vi "BTS_PWMTest_GDCB-7_v1.vi"(8 "error in (no error)":errorcluster, 10 "HMP VISA":refnum<visa-resource-name>, 11 "ControlBoard VISA":refnum<visa-resource-name>) -> (0 "error out":errorcluster, 2 "Message OUT":string, 3 "Result (bool)":bool)   [LabVIEW 2022 SP3]
uses:
  HMP4000 Communication/HMP4040_ChannelControlAutomatic.ctl
  <vilib>/DAQmx/read.llb/DAQmx Read (Analog 1D Wfm NChan NSamp).vi
  <vilib>/DAQmx/miscellaneous.llb/DAQmx Fill In Error Info.vi
panel:
  in  "Message IN":string=" "
  out "Analysis Leg":i32
  out "Waveforms":T1
  out "Active Leg":i32
  out "Result (color)":u32(colorbox)
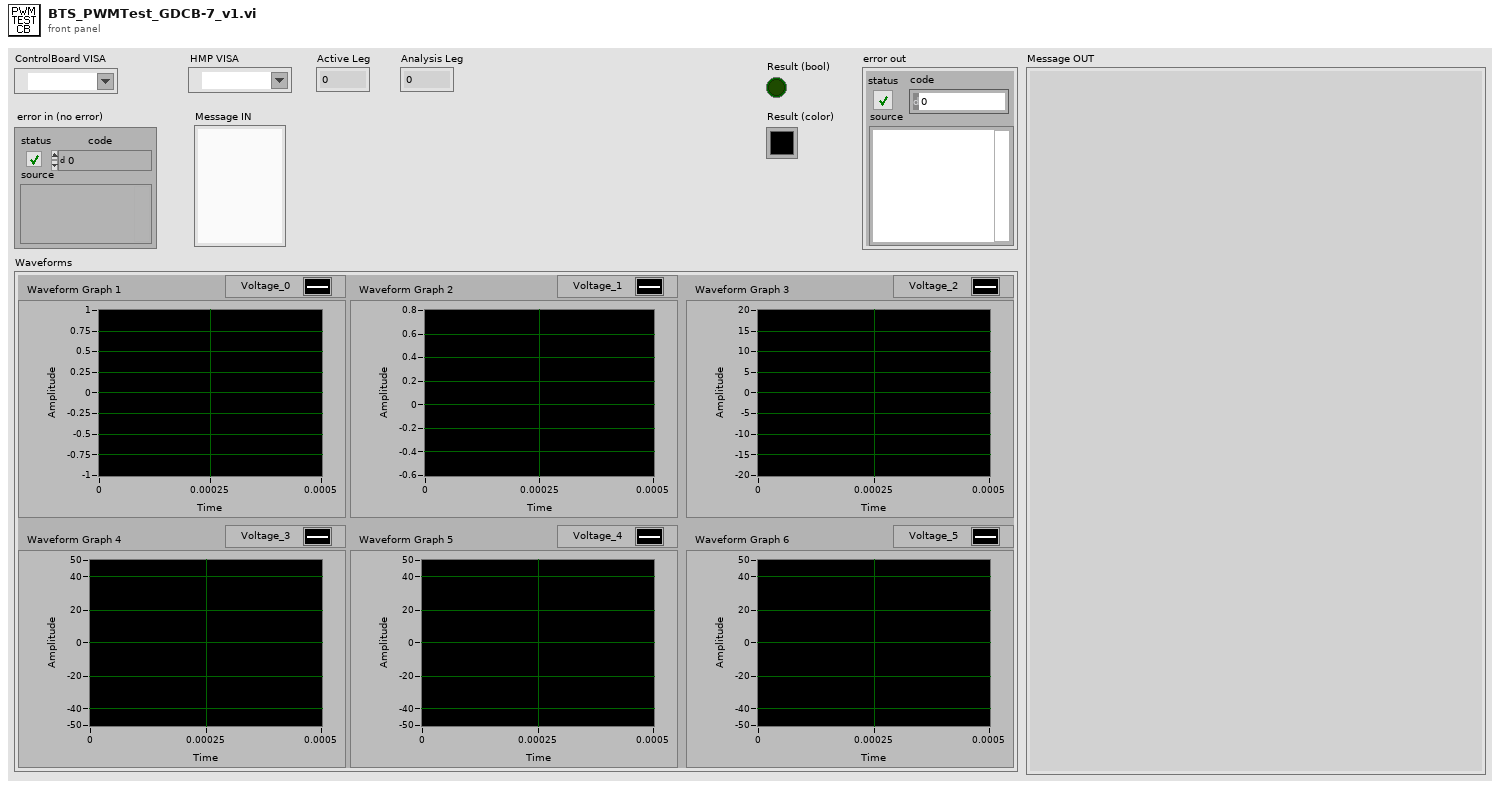
[diagram p1: front panel]
types:
  T1 = cluster{"Waveform Graph 1":waveform(dbl), "Waveform Graph 2":waveform(dbl), "Waveform Graph 3":waveform(dbl), "Waveform Graph 4":waveform(dbl), "Waveform Graph 5":waveform(dbl), "Waveform Graph 6":waveform(dbl)}
  T2 = typedef "HMP4040_ChannelControlAutomatic.ctl" = enum16{"Off", "Control Power", "HMP2020 Control + DC32V", "HMP2020 Control + DC8V", "HMP4040 Control + DC32V", "HMP4040 Control +DC8V", "HMP4040 Ch2 24V 4A"}
  T3 = cluster{"data[0]":waveform(dbl), "data[1]":waveform(dbl), "data[2]":waveform(dbl), "data[3]":waveform(dbl), "data[4]":waveform(dbl), "data[5]":waveform(dbl)}
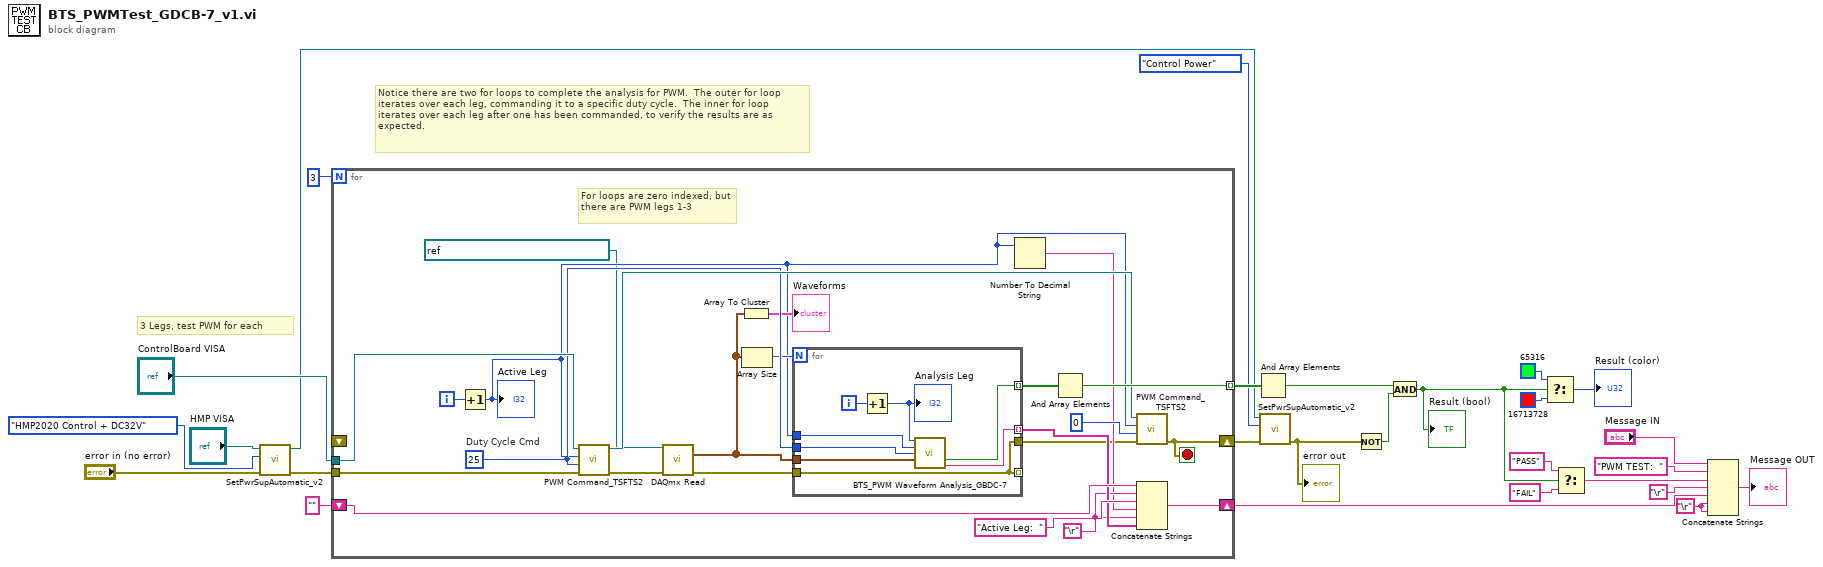
[diagram p0: block diagram]
diagram:
  w17 = "\r"
  # "Notice there are two for loops to complete the analysis for PWM.  The outer for loop iterates over each leg, commanding it to a specific duty cycle.  The inner for loop iterates over each leg after one has been commanded, to verify the results are as expected."
  # "3 Legs, test PWM for each"
  n1 = call "SetPwrSupAutomatic_v2.vi"("error in (no error)"="error in (no error)", "Enum"=HMP4040_ChannelControlAutomatic."HMP2020 Control + DC32V", "HMP VISA"="HMP VISA") -> ("error out"=w1:errorcluster, "HMP VISA Out"=w5:refnum<visa-resource-name>)  [unwired: 7 in]
  n2 = for {
    N: 3 -> [_]
    tunnel: "ControlBoard VISA" -> [w45]
    tunnel: [w50] -> w27 mode=indexing
    shift-right: [w49] -> w15
    shift-left: "" -> [w48]
    shift-right: [w31] -> w9
    shift-left: _ -> [_]
    tunnel: w1 -> [w29]
    i -> [w43]
    stop <- w31 stop-if-true
    w34 = "\r"
    w44 = 25  # Duty Cycle Cmd
    # "For loops are zero indexed, but there are PWM legs 1-3"
    n3 = Increment(x=w43) -> (x+1=w36:i32)
    "Active Leg" <- w36
    n4 = call "PWM Command_TSFTS2.vi"("error in (no error)"=w29, "Duty Cycle"=w44, "Leg"=w36, "VISA Refnum in"=w45) -> ("error out"=w38:errorcluster, "VISA Refnum out"=w46:refnum<visa-resource-name>)  [unwired: 5 in, 1 out]
    n5 = call-poly <vilib>:"DAQmx Read.vi"("task/channels in"=refnum<k21> "BTS_PWMInput_CarrierBoard", "error in"=w38) -> ("data"=w39:waveform(dbl)[], "error out"=w32:errorcluster)  [unwired: 11 in, 1 out]
    n6 = Array To Cluster(array=w39) -> (cluster=→"Waveforms":T3)
    n7 = Array Size(array=w39) -> (size(s)=w40:i32)
    n8 = for {
      N: w40 -> [_]
      tunnel: w44 -> [w58]
      tunnel: w39 -> [w57]
      tunnel: w36 -> [w56]
      tunnel: [w53] -> w41 mode=indexing
      tunnel: [w52] -> w35 mode=indexing
      tunnel: w32 -> [w51]
      tunnel: [w51] -> _ mode=indexing
      tunnel: [w51] -> w30
      i -> [w55]
      n9 = Increment(x=w55) -> (x+1=w54:i32)
      "Analysis Leg" <- w54
      n10 = call "BTS_PWM Waveform Analysis_GBDC-7.vi"("Analysis Leg"=w54, "Active Leg"=w56, "Duty Cycle"=w58, "Waveform"=w57) -> ("Result (Boolean)"=w53:bool, "Message"=w52:string)  [unwired: 9 in, 1 out]
    }
    n11 = Number To Decimal String(number=w36) -> (decimal integer string=w33:string)  [unwired: 1 in]
    n12 = And Array Elements(Boolean array=w41) -> (logical AND=w50:bool)
    n13 = call "PWM Command_TSFTS2.vi"("error in (no error)"=w30, "Duty Cycle"=0, "Leg"=w36, "VISA Refnum in"=w46) -> ("error out"=w31:errorcluster)  [unwired: 5 in, 2 out]
    n14 = Concatenate Strings(w48, w34, "Active Leg:  ", w33, w34, w35) -> (w49:string)
  }
  n15 = And Array Elements(Boolean array=w27) -> (logical AND=w18:bool)
  n16 = call "SetPwrSupAutomatic_v2.vi"("error in (no error)"=w9, "Enum"=HMP4040_ChannelControlAutomatic."Control Power", "HMP VISA"=w5) -> ("error out"=w2:errorcluster)  [unwired: 7 in, 1 out]
  "error out" <- w2
  n17 = Not(x=w2) -> (.not. x?=w20:bool)
  n18 = And(x=w18, y=w20) -> (x .and. y?=w19:bool)
  "Result (bool)" <- w19
  n19 = Select(t=u32 65316 ("Result (color)"), s=w19, f=u32 16713728 ("Result (color)")) -> (s? t:f=→"Result (color)":u32)
  n20 = Select(t="PASS", s=w19, f="FAIL") -> (s? t:f=w10:string)
  n21 = Concatenate Strings("Message IN", "PWM TEST:  ", w10, "\r", w15, w17, w17) -> (→"Message OUT":string)
